vi "Match Regex.vi"(8 "error in (no error)":errorcluster, 9 "Exclude? (F)":bool, 10 "regular expression":string, 11 "Labels":string[](array[string])) -> (0 "error out":errorcluster, 3 "Array":string[](array[string]))   [LabVIEW 2023, in "Label-Driven UI.lvlib"]
uses:
  Label-Driven UI.lvlib
  <vilib>/regexp/Match Regular Expression.xnode
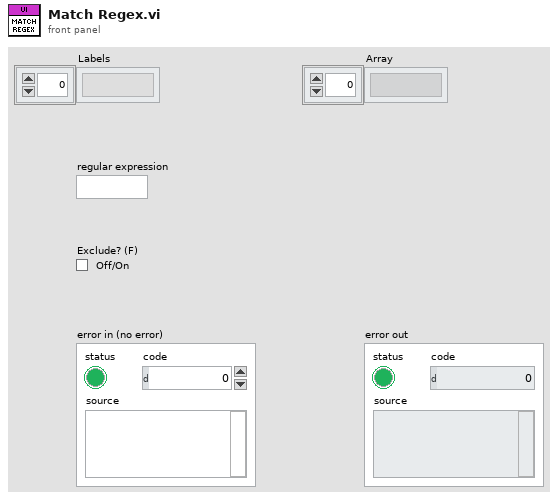
[diagram p1: front panel]
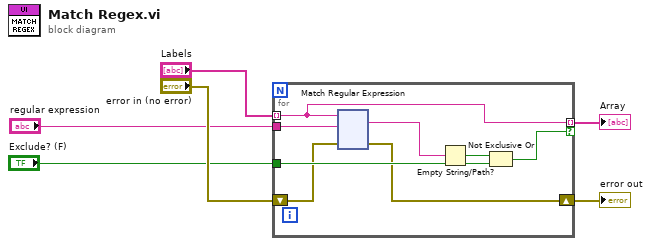
[diagram p0: block diagram]
diagram:
  n1 = for {
    tunnel: "Labels" -> [w7] mode=indexing
    tunnel: "regular expression" -> [w14]
    tunnel: [w7] -> w6 mode=indexing if=w10
    tunnel: "Exclude? (F)" -> [w11]
    shift-right: [w8] -> w5
    shift-left: "error in (no error)" -> [w9]
    n2 = xnode "Match Regular Expression"("input string"=w7, "regular expression"=w14, "error in"=w9) -> ("whole match"=w13:string, "error out"=w8:errorcluster)  [unwired: 3 in, 3 out]
    n3 = Empty String/Path?(string/path=w13) -> (empty?=w12:bool)
    n4 = Not Exclusive Or(1:w11, 2:w12) -> (0:w10:bool)
  }
  "Array" <- w6
  "error out" <- w5
